vi "Write Message Status.vi"(8 "error in (no error)":errorcluster, 10 "Message Status":T1 items=["Simple", "Dialog", "PVUpdate", "Dialog + PVUpdate", "N/A"], 11 "CS++Message in":refnum<class "CS++Message.lvclass">) -> (0 "error out":errorcluster, 3 "CS++Message out":refnum<class "CS++Message.lvclass">)   [LabVIEW 2015, in "CS++Message.lvlib" / "CS++Message.lvclass"]
uses:
  CS++Message.lvclass
  MessageStatus.ctl
  CS++Message.lvclass/CS++Message.ctl
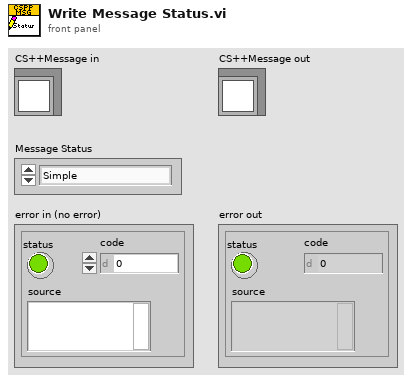
[diagram p1: front panel]
types:
  T1 = typedef "CS++Message.lvlib/CS++Message.lvclass/MessageStatus.ctl" = u16
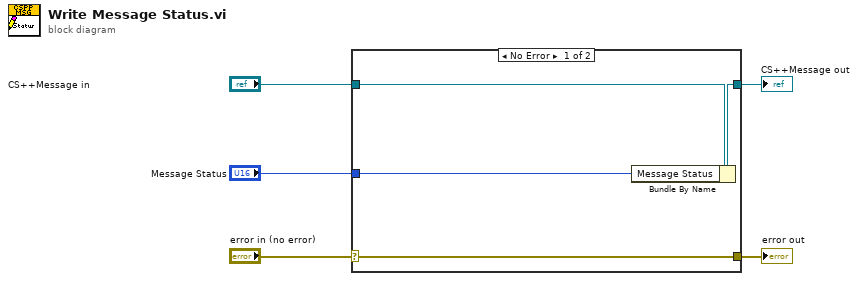
[diagram p0: block diagram]
diagram:
  n1 = case shown="No Error" "error in (no error)" {
    selector: "error in (no error)" -> [w9 w10]
    tunnel: [w9 w10] -> w4
    tunnel: [w7 w11] -> w2
    tunnel: "CS++Message in" -> [w8 w11]
    tunnel: "Message Status" -> [w6 _]
    frame No Error {
      n2 = Bundle By Name(cluster=w8, "Message Status"=w6) -> (w7:refnum<class "CS++Message.lvclass">)
    }
    frame Error {
    }
  }
  "error out" <- w4
  "CS++Message out" <- w2
